vi "setState.vi"(0 "Interface in":T2, 5 "PI_Controller":T1, 7 "PI_state":enum8{"idle", "normal", "manual", "perturbance"}(ring), 9 "manual":sgl format="%#_13g", 11 "error in":errorcluster, 12 "reset":bool) -> (4 "Interface out":T2, 15 "error out":errorcluster)   [LabVIEW 2017, in "AFE_interface.lvlib"]
uses:
  AFE_interface.lvlib
  InterfaceRef.ctl
  <instrlib>/_niInstr/Instruction Framework/v1/Host/Instruction Target/niInstr Instruction Target v1 Host.lvclass
  <instrlib>/_niInstr/Instruction Framework/v1/Host/Instruction Framework Context/niInstr Instruction Framework Context v1 Host.lvclass
  PI_Controllers.ctl
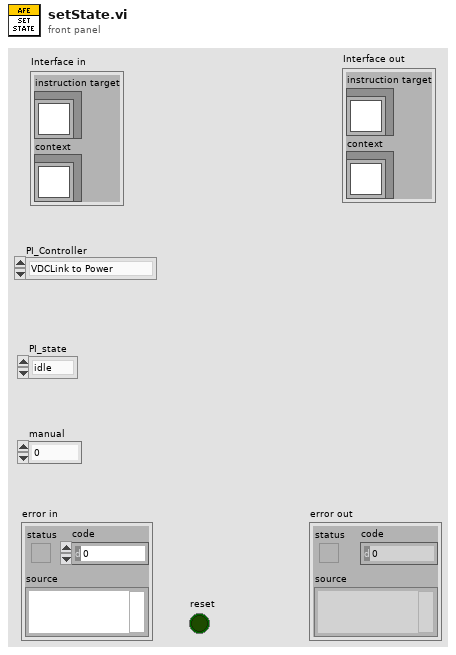
[diagram p1: front panel]
types:
  T1 = typedef "AFE_interface.lvlib/PI_Controllers.ctl" = enum16{"VDCLink to Power", "ID to VD", "IQ to VQ"}
  T2 = typedef "AFE_interface.lvlib/InterfaceRef.ctl" = cluster{"instruction target":refnum<class "niInstr Instruction Target v1 Host.lvclass">, "context":refnum<class "niInstr Instruction Framework Context v1 Host.lvclass">}
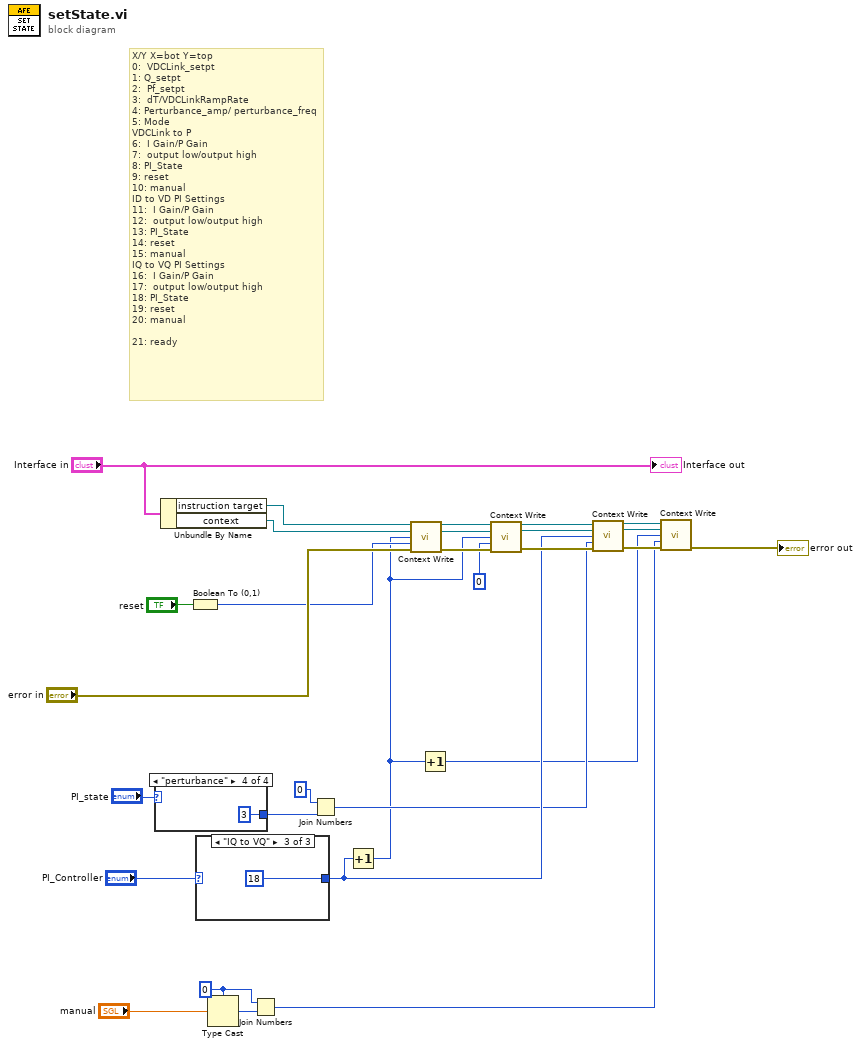
[diagram p0: block diagram]
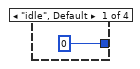
[diagram p2: hidden frame]
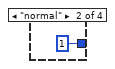
[diagram p3: hidden frame]
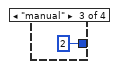
[diagram p4: hidden frame]
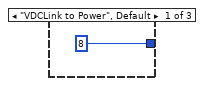
[diagram p5: hidden frame]
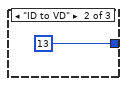
[diagram p6: hidden frame]
diagram:
  w10 = u32 0
  # "X/Y X=bot Y=top\n0:  VDCLink_setpt\n1: Q_setpt\n2:  Pf_setpt\n3:  dT/VDCLinkRampRate\n4: Perturbance_amp/ perturbance_freq\n5: Mode\nVDCLink to P\n6:  I Gain/P Gain\n7:  output low/output high\n8: PI_State\n9: reset\n10: manual\nID to VD PI Settings \n11:  I Gain/P Gain\n12:  output low/output high\n13: PI_State\n14: reset\n15: manual\nIQ to VQ PI Settings\n16:  I Gain/P Gain\n17:  output low/output high\n18: PI_State\n19: reset\n20: manual\n\n21: ready"
  n1 = case shown="\"perturbance\"" "PI_state" {
    tunnel: [u32 0 ("hi") u32 1 ("hi") u32 2 ("hi") u32 3 ("hi")] -> w1
    frame "idle", Default {
    }
    frame "normal" {
    }
    frame "manual" {
    }
    frame "perturbance" {
    }
  }
  n2 = Unbundle By Name("Interface in") -> ("instruction target"=w19:refnum<class "niInstr Instruction Target v1 Host.lvclass">, "context"=w20:refnum<class "niInstr Instruction Framework Context v1 Host.lvclass">)
  n3 = Boolean To (0,1)(Boolean="reset") -> (0, 1=w15:i16)
  n4 = case shown="\"IQ to VQ\"" "PI_Controller" {
    tunnel: [8 ("y") 13 ("y") 18 ("y")] -> w18
    frame "VDCLink to Power", Default {
    }
    frame "ID to VD" {
    }
    frame "IQ to VQ" {
    }
  }
  n5 = Type Cast(type=w10, x="manual") -> (*(type *) &x=w11:u32)
  n6 = Join Numbers(hi=w10, lo=w11) -> ((hi.lo)=w3:u64)
  n7 = Join Numbers(hi=u32 0, lo=w1) -> ((hi.lo)=w12:u64)
  n8 = Increment(x=w18) -> (x+1=w5:i32)
  n9 = call <instrlib>:"Context Write.vi"("instruction target in"=w19, "context in"=w20, "address"=w5, "data"=w15, "error in"="error in") -> ("instruction target out"=w23:refnum<class "niInstr Instruction Target v1 Host.lvclass">, "context out"=w21:refnum<class "niInstr Instruction Framework Context v1 Host.lvclass">, "error out"=w22:errorcluster)  [unwired: 8 in]
  n10 = Increment(x=w5) -> (x+1=w4:i32)
  n11 = call <instrlib>:"Context Write.vi"("instruction target in"=w23, "context in"=w21, "address"=w5, "data"=u64 0, "error in"=w22) -> ("instruction target out"=w28:refnum<class "niInstr Instruction Target v1 Host.lvclass">, "context out"=w26:refnum<class "niInstr Instruction Framework Context v1 Host.lvclass">, "error out"=w27:errorcluster)  [unwired: 8 in]
  n12 = call <instrlib>:"Context Write.vi"("instruction target in"=w28, "context in"=w26, "address"=w18, "data"=w12, "error in"=w27) -> ("instruction target out"=w9:refnum<class "niInstr Instruction Target v1 Host.lvclass">, "context out"=w7:refnum<class "niInstr Instruction Framework Context v1 Host.lvclass">, "error out"=w8:errorcluster)  [unwired: 8 in]
  n13 = call <instrlib>:"Context Write.vi"("instruction target in"=w9, "context in"=w7, "address"=w4, "data"=w3, "error in"=w8) -> ("error out"=→"error out":errorcluster)  [unwired: 8 in, 2 out]
  "Interface out" <- "Interface in"
